vi "rsidr_core_global.vi"() -> ()   [LabVIEW 2020, in "Rohde&Schwarz CMWXP NR FR1 Measurement.lvlib"] (continued)
"Descriptive Name"="Query Multi Eval Meas List EVM DMRS Low Current Limit Check Results", "Data Type"=enum."RawString", "Command"="CALC:NRS:MEAS{instance}:MEV:LIST:MOD:EVM:DMRS:LOW:CURR?", "Access"=enum."Read Only", "Range Table"="", "Read Callback"="", "Write Callback"="", "Range Callback"="", "Check Callback"="", "Rngtable Callback"="", "Coerce Callback"="", "Supported Models"="", "Instrument Options"="", "Check Status Callback"="", "Flags"=0, "Help"="Return error vector magnitude DMRS limit check results for low EVM window position, for all measured list mode segments.\n\nReturn values:  \n<Reliability>\n decimal\n\n<EVM_DMRSLimCheck>\n limit check result\nComma-separated list of values, one per measured segment\nDefault unit:  %\n\nAvailable Repeated Capabilities:\ninstance: i0, i1, i2, i3, i4, i5, i6, i7, i8, i9, i10, i11, i12, i13, i14, i15, i16, i17, i18, i19, i20, i21, i22, i23, i24, i25, i26, i27, i28, i29, i30, i31, i32\r\n\nRemote-control command(s):\nCALCulate:NRSub:MEAS<i>:MEValuation:LIST:MODulation:EVM:DMRS:LOW:CURRent?"}, {"Level"=5, "Class Only"=FALSE, "Identifier"="RSCMWXPNRFR1M_ATTR_QUERY_MULTI_EVAL_MEAS_LIST_EVM_DMRS_LOW_AVERAGE_LIMIT_CHECK_RESULTS", "Descriptive Name"="Query Multi Eval Meas List EVM DMRS Low Average Limit Check Results", "Data Type"=enum."RawString", "Command"="CALC:NRS:MEAS{instance}:MEV:LIST:MOD:EVM:DMRS:LOW:AVER?", "Access"=enum."Read Only", "Range Table"="", "Read Callback"="", "Write Callback"="", "Range Callback"="", "Check Callback"="", "Rngtable Callback"="", "Coerce Callback"="", "Supported Models"="", "Instrument Options"="", "Check Status Callback"="", "Flags"=0, "Help"="Return average error vector magnitude DMRS limit check results for low EVM window position, for all measured list mode segments.\n\nReturn values:  \n<Reliability>\n decimal\n\n<EVM_DMRSLimCheck>\n limit check result\nComma-separated list of values, one per measured segment\nDefault unit:  %\n\nAvailable Repeated Capabilities:\ninstance: i0, i1, i2, i3, i4, i5, i6, i7, i8, i9, i10, i11, i12, i13, i14, i15, i16, i17, i18, i19, i20, i21, i22, i23, i24, i25, i26, i27, i28, i29, i30, i31, i32\r\n\nRemote-control command(s):\nCALCulate:NRSub:MEAS<i>:MEValuation:LIST:MODulation:EVM:DMRS:LOW:AVERage?"}, {"Level"=5, "Class Only"=FALSE, "Identifier"="RSCMWXPNRFR1M_ATTR_QUERY_MULTI_EVAL_MEAS_LIST_EVM_DMRS_LOW_EXTREME_LIMIT_CHECK_RESULTS", "Descriptive Name"="Query Multi Eval Meas List EVM DMRS Low Extreme Limit Check Results", "Data Type"=enum."RawString", "Command"="CALC:NRS:MEAS{instance}:MEV:LIST:MOD:EVM:DMRS:LOW:EXTR?", "Access"=enum."Read Only", "Range Table"="", "Read Callback"="", "Write Callback"="", "Range Callback"="", "Check Callback"="", "Rngtable Callback"="", "Coerce Callback"="", "Supported Models"="", "Instrument Options"="", "Check Status Callback"="", "Flags"=0, "Help"="Return extreme error vector magnitude DMRS limit check results for low EVM window position, for all measured list mode segments.\n\nReturn values:  \n<Reliability>\n decimal\n\n<EVM_DMRSLimCheck>\n limit check result\nComma-separated list of values, one per measured segment\nDefault unit:  %\n\nAvailable Repeated Capabilities:\ninstance: i0, i1, i2, i3, i4, i5, i6, i7, i8, i9, i10, i11, i12, i13, i14, i15, i16, i17, i18, i19, i20, i21, i22, i23, i24, i25, i26, i27, i28, i29, i30, i31, i32\r\n\nRemote-control command(s):\nCALCulate:NRSub:MEAS<i>:MEValuation:LIST:MODulation:EVM:DMRS:LOW:EXTReme?"}, {"Level"=5, "Class Only"=FALSE, "Identifier"="RSCMWXPNRFR1M_ATTR_QUERY_MULTI_EVAL_MEAS_LIST_EVM_DMRS_HIGH_CURRENT_LIMIT_CHECK_RESULTS", "Descriptive Name"="Query Multi Eval Meas List EVM DMRS High Current Limit Check Results", "Data Type"=enum."RawString", "Command"="CALC:NRS:MEAS{instance}:MEV:LIST:MOD:EVM:DMRS:HIGH:CURR?", "Access"=enum."Read Only", "Range Table"="", "Read Callback"="", "Write Callback"="", "Range Callback"="", "Check Callback"="", "Rngtable Callback"="", "Coerce Callback"="", "Supported Models"="", "Instrument Options"="", "Check Status Callback"="", "Flags"=0, "Help"="Return error vector magnitude DMRS limit check results for high EVM window position, for all measured list mode segments.\n\nReturn values:  \n<Reliability>\n decimal\n\n<EVM_DMRSLimCheck>\n limit check result\nComma-separated list of values, one per measured segment\nDefault unit:  %\n\nAvailable Repeated Capabilities:\ninstance: i0, i1, i2, i3, i4, i5, i6, i7, i8, i9, i10, i11, i12, i13, i14, i15, i16, i17, i18, i19, i20, i21, i22, i23, i24, i25, i26, i27, i28, i29, i30, i31, i32\r\n\nRemote-control command(s):\nCALCulate:NRSub:MEAS<i>:MEValuation:LIST:MODulation:EVM:DMRS:HIGH:CURRent?"}, {"Level"=5, "Class Only"=FALSE, "Identifier"="RSCMWXPNRFR1M_ATTR_QUERY_MULTI_EVAL_MEAS_LIST_EVM_DMRS_HIGH_AVERAGE_LIMIT_CHECK_RESULTS", "Descriptive Name"="Query Multi Eval Meas List EVM DMRS High Average Limit Check Results", "Data Type"=enum."RawString", "Command"="CALC:NRS:MEAS{instance}:MEV:LIST:MOD:EVM:DMRS:HIGH:AVER?", "Access"=enum."Read Only", "Range Table"="", "Read Callback"="", "Write Callback"="", "Range Callback"="", "Check Callback"="", "Rngtable Callback"="", "Coerce Callback"="", "Supported Models"="", "Instrument Options"="", "Check Status Callback"="", "Flags"=0, "Help"="Return average error vector magnitude DMRS limit check results for high EVM window position, for all measured list mode segments.\n\nReturn values:  \n<Reliability>\n decimal\n\n<EVM_DMRSLimCheck>\n limit check result\nComma-separated list of values, one per measured segment\nDefault unit:  %\n\nAvailable Repeated Capabilities:\ninstance: i0, i1, i2, i3, i4, i5, i6, i7, i8, i9, i10, i11, i12, i13, i14, i15, i16, i17, i18, i19, i20, i21, i22, i23, i24, i25, i26, i27, i28, i29, i30, i31, i32\r\n\nRemote-control command(s):\nCALCulate:NRSub:MEAS<i>:MEValuation:LIST:MODulation:EVM:DMRS:HIGH:AVERage?"}, {"Level"=5, "Class Only"=FALSE, "Identifier"="RSCMWXPNRFR1M_ATTR_QUERY_MULTI_EVAL_MEAS_LIST_EVM_DMRS_HIGH_EXTREME_LIMIT_CHECK_RESULTS", "Descriptive Name"="Query Multi Eval Meas List EVM DMRS High Extreme Limit Check Results", "Data Type"=enum."RawString", "Command"="CALC:NRS:MEAS{instance}:MEV:LIST:MOD:EVM:DMRS:HIGH:EXTR?", "Access"=enum."Read Only", "Range Table"="", "Read Callback"="", "Write Callback"="", "Range Callback"="", "Check Callback"="", "Rngtable Callback"="", "Coerce Callback"="", "Supported Models"="", "Instrument Options"="", "Check Status Callback"="", "Flags"=0, "Help"="Return extreme error vector magnitude DMRS limit check results for high EVM window position, for all measured list mode segments.\n\nReturn values:  \n<Reliability>\n decimal\n\n<EVM_DMRSLimCheck>\n limit check result\nComma-separated list of values, one per measured segment\nDefault unit:  %\n\nAvailable Repeated Capabilities:\ninstance: i0, i1, i2, i3, i4, i5, i6, i7, i8, i9, i10, i11, i12, i13, i14, i15, i16, i17, i18, i19, i20, i21, i22, i23, i24, i25, i26, i27, i28, i29, i30, i31, i32\r\n\nRemote-control command(s):\nCALCulate:NRSub:MEAS<i>:MEValuation:LIST:MODulation:EVM:DMRS:HIGH:EXTReme?"}, {"Level"=4, "Class Only"=TRUE, "Identifier"="", "Descriptive Name"="Inband Emission", "Data Type"=enum."ViInt32", "Command"="", "Access"=enum."Read Only", "Range Table"="", "Read Callback"="", "Write Callback"="", "Range Callback"="", "Check Callback"="", "Rngtable Callback"="", "Coerce Callback"="", "Supported Models"="", "Instrument Options"="", "Check Status Callback"="", "Flags"=0, "Help"="The attributes in this class return inband emission limit line margin results for all measured segments. The number of returned results depends on the number of measured segments."}, {"Level"=5, "Class Only"=FALSE, "Identifier"="RSCMWXPNRFR1M_ATTR_FETCH_MULTI_EVAL_MEAS_LIST_IEM_MARGIN_CURRENT_RESULTS", "Descriptive Name"="Fetch Multi Eval Meas List IEM Margin Current Results", "Data Type"=enum."RawString", "Command"="FETC:NRS:MEAS{instance}:MEV:LIST:IEM:MARG:CURR?", "Access"=enum."Read Only", "Range Table"="", "Read Callback"="", "Write Callback"="", "Range Callback"="", "Check Callback"="", "Rngtable Callback"="", "Coerce Callback"="", "Supported Models"="", "Instrument Options"="", "Check Status Callback"="", "Flags"=0, "Help"="Return the inband emission limit line margin results for all measured list mode segments. The current margins indicate the minimum (vertical) distance between the limit line and the current trace. A negative result indicates that the limit is exceeded. The average, extreme and standard deviation values are calculated from the current margins.\n\nThe results are returned as triplets per segment: <Reliability>, {<Margin>, <IQImage>, <CarrLeakage>}seg 1, {<Margin>, <IQImage>, <CarrLeakage>}seg 2, ...\n\nReturn values:  \n<Reliability>\n decimal\n\n<Margin>\n float\nMargin over all non-allocated RBs (scope of general limit component)\nDefault unit:  dB \n\n<IQImage>\n float\nMargin at image frequencies of allocated RBs (scope of IQ image limit component)\nDefault unit:  dB \n\n<CarrLeakage>\n float\nMargin at the carrier frequency (scope of IQ offset limit component)\nDefault unit:  dB\n\nAvailable Repeated Capabilities:\ninstance: i0, i1, i2, i3, i4, i5, i6, i7, i8, i9, i10, i11, i12, i13, i14, i15, i16, i17, i18, i19, i20, i21, i22, i23, i24, i25, i26, i27, i28, i29, i30, i31, i32\r\n\nRemote-control command(s):\nFETCh:NRSub:MEAS<i>:MEValuation:LIST:IEMission:MARGin:CURRent?"}, {"Level"=5, "Class Only"=FALSE, "Identifier"="RSCMWXPNRFR1M_ATTR_FETCH_MULTI_EVAL_MEAS_LIST_IEM_MARGIN_AVERAGE_RESULTS", "Descriptive Name"="Fetch Multi Eval Meas List IEM Margin Average Results", "Data Type"=enum."RawString", "Command"="FETC:NRS:MEAS{instance}:MEV:LIST:IEM:MARG:AVER?", "Access"=enum."Read Only", "Range Table"="", "Read Callback"="", "Write Callback"="", "Range Callback"="", "Check Callback"="", "Rngtable Callback"="", "Coerce Callback"="", "Supported Models"="", "Instrument Options"="", "Check Status Callback"="", "Flags"=0, "Help"="Return the average inband emission limit line margin results for all measured list mode segments. The current margins indicate the minimum (vertical) distance between the limit line and the current trace. A negative result indicates that the limit is exceeded. The average, extreme and standard deviation values are calculated from the current margins.\n\nThe results are returned as triplets per segment: <Reliability>, {<Margin>, <IQImage>, <CarrLeakage>}seg 1, {<Margin>, <IQImage>, <CarrLeakage>}seg 2, ...\n\nReturn values:  \n<Reliability>\n decimal\n\n<Margin>\n float\nMargin over all non-allocated RBs (scope of general limit component)\nDefault unit:  dB \n\n<IQImage>\n float\nMargin at image frequencies of allocated RBs (scope of IQ image limit component)\nDefault unit:  dB \n\n<CarrLeakage>\n float\nMargin at the carrier frequency (scope of IQ offset limit component)\nDefault unit:  dB\n\nAvailable Repeated Capabilities:\ninstance: i0, i1, i2, i3, i4, i5, i6, i7, i8, i9, i10, i11, i12, i13, i14, i15, i16, i17, i18, i19, i20, i21, i22, i23, i24, i25, i26, i27, i28, i29, i30, i31, i32\r\n\nRemote-control command(s):\nFETCh:NRSub:MEAS<i>:MEValuation:LIST:IEMission:MARGin:AVERage?"}, {"Level"=5, "Class Only"=FALSE, "Identifier"="RSCMWXPNRFR1M_ATTR_FETCH_MULTI_EVAL_MEAS_LIST_IEM_MARGIN_EXTREME_RESULTS", "Descriptive Name"="Fetch Multi Eval Meas List IEM Margin Extreme Results", "Data Type"=enum."RawString", "Command"="FETC:NRS:MEAS{instance}:MEV:LIST:IEM:MARG:EXTR?", "Access"=enum."Read Only", "Range Table"="", "Read Callback"="", "Write Callback"="", "Range Callback"="", "Check Callback"="", "Rngtable Callback"="", "Coerce Callback"="", "Supported Models"="", "Instrument Options"="", "Check Status Callback"="", "Flags"=0, "Help"="Return the extreme inband emission limit line margin results for all measured list mode segments. The current margins indicate the minimum (vertical) distance between the limit line and the current trace. A negative result indicates that the limit is exceeded. The average, extreme and standard deviation values are calculated from the current margins.\n\nThe results are returned as triplets per segment: <Reliability>, {<Margin>, <IQImage>, <CarrLeakage>}seg 1, {<Margin>, <IQImage>, <CarrLeakage>}seg 2, ...\n\nReturn values:  \n<Reliability>\n decimal\n\n<Margin>\n float\nMargin over all non-allocated RBs (scope of general limit component)\nDefault unit:  dB \n\n<IQImage>\n float\nMargin at image frequencies of allocated RBs (scope of IQ image limit component)\nDefault unit:  dB \n\n<CarrLeakage>\n float\nMargin at the carrier frequency (scope of IQ offset limit component)\nDefault unit:  dB\n\nAvailable Repeated Capabilities:\ninstance: i0, i1, i2, i3, i4, i5, i6, i7, i8, i9, i10, i11, i12, i13, i14, i15, i16, i17, i18, i19, i20, i21, i22, i23, i24, i25, i26, i27, i28, i29, i30, i31, i32\r\n\nRemote-control command(s):\nFETCh:NRSub:MEAS<i>:MEValuation:LIST:IEMission:MARGin:EXTReme?"}, {"Level"=5, "Class Only"=FALSE, "Identifier"="RSCMWXPNRFR1M_ATTR_FETCH_MULTI_EVAL_MEAS_LIST_IEM_MARGIN_STANDARD_DEVIATION_RESULTS", "Descriptive Name"="Fetch Multi Eval Meas List IEM Margin Standard Deviation Results", "Data Type"=enum."RawString", "Command"="FETC:NRS:MEAS{instance}:MEV:LIST:IEM:MARG:SDEV?", "Access"=enum."Read Only", "Range Table"="", "Read Callback"="", "Write Callback"="", "Range Callback"="", "Check Callback"="", "Rngtable Callback"="", "Coerce Callback"="", "Supported Models"="", "Instrument Options"="", "Check Status Callback"="", "Flags"=0, "Help"="Return the standard deviation inband emission limit line margin results for all measured list mode segments. The current margins indicate the minimum (vertical) distance between the limit line and the current trace. A negative result indicates that the limit is exceeded. The average, extreme and standard deviation values are calculated from the current margins.\n\nThe results are returned as triplets per segment: <Reliability>, {<Margin>, <IQImage>, <CarrLeakage>}seg 1, {<Margin>, <IQImage>, <CarrLeakage>}seg 2, ...\n\nReturn values:  \n<Reliability>\n decimal\n\n<Margin>\n float\nMargin over all non-allocated RBs (scope of general limit component)\nDefault unit:  dB \n\n<IQImage>\n float\nMargin at image frequencies of allocated RBs (scope of IQ image limit component)\nDefault unit:  dB \n\n<CarrLeakage>\n float\nMargin at the carrier frequency (scope of IQ offset limit component)\nDefault unit:  dB\n\nAvailable Repeated Capabilities:\ninstance: i0, i1, i2, i3, i4, i5, i6, i7, i8, i9, i10, i11, i12, i13, i14, i15, i16, i17, i18, i19, i20, i21, i22, i23, i24, i25, i26, i27, i28, i29, i30, i31, i32\r\n\nRemote-control command(s):\nFETCh:NRSub:MEAS<i>:MEValuation:LIST:IEMission:MARGin:SDEViation?"}, {"Level"=5, "Class Only"=FALSE, "Identifier"="RSCMWXPNRFR1M_ATTR_FETCH_MULTI_EVAL_MEAS_LIST_IEM_MARGIN_RB_INDEX_CURRENT_RESULTS", "Descriptive Name"="Fetch Multi Eval Meas List IEM Margin RB Index Current Results", "Data Type"=enum."RawString", "Command"="FETC:NRS:MEAS{instance}:MEV:LIST:IEM:MARG:CURR:RBIN?", "Access"=enum."Read Only", "Range Table"="", "Read Callback"="", "Write Callback"="", "Range Callback"="", "Check Callback"="", "Rngtable Callback"="", "Coerce Callback"="", "Supported Models"="", "Instrument Options"="", "Check Status Callback"="", "Flags"=0, "Help"="Return resource block indices of the inband emission measurement for all measured list mode segments. At these RB indices, the current margins have been detected.\n\nThe results are returned as triplets per segment: <Reliability>, {<RBindex>, <IQImage>, <CarrLeakage>}seg 1, {<RBindex>, <IQImage>, <CarrLeakage>}seg 2, ...\n\nReturn values:  \n<Reliability>\n decimal\n\n<RBindex>\n decimal\nResource block index for the general margin (at non-allocated RBs)\n\n<IQImage>\n decimal\nResource block index for the IQ image margin (at image frequencies of allocated RBs)\n\n<CarrLeakage>\n decimal\nResource block index for the carrier leakage margin (at carrier frequency)\n\nAvailable Repeated Capabilities:\ninstance: i0, i1, i2, i3, i4, i5, i6, i7, i8, i9, i10, i11, i12, i13, i14, i15, i16, i17, i18, i19, i20, i21, i22, i23, i24, i25, i26, i27, i28, i29, i30, i31, i32\r\n\nRemote-control command(s):\nFETCh:NRSub:MEAS<i>:MEValuation:LIST:IEMission:MARGin:CURRent:RBINdex?"}, {"Level"=5, "Class Only"=FALSE, "Identifier"="RSCMWXPNRFR1M_ATTR_FETCH_MULTI_EVAL_MEAS_LIST_IEM_MARGIN_RB_INDEX_AVERAGE_RESULTS", "Descriptive Name"="Fetch Multi Eval Meas List IEM Margin RB Index Average Results", "Data Type"=enum."RawString", "Command"="FETC:NRS:MEAS{instance}:MEV:LIST:IEM:MARG:AVER:RBIN?", "Access"=enum."Read Only", "Range Table"="", "Read Callback"="", "Write Callback"="", "Range Callback"="", "Check Callback"="", "Rngtable Callback"="", "Coerce Callback"="", "Supported Models"="", "Instrument Options"="", "Check Status Callback"="", "Flags"=0, "Help"="Return resource block indices of the inband emission measurement for all measured list mode segments. At these RB indices, the average margins have been detected.\n\nThe results are returned as triplets per segment: <Reliability>, {<RBindex>, <IQImage>, <CarrLeakage>}seg 1, {<RBindex>, <IQImage>, <CarrLeakage>}seg 2, ...\n\nReturn values:  \n<Reliability>\n decimal\n\n<RBindex>\n decimal\nResource block index for the general margin (at non-allocated RBs)\n\n<IQImage>\n decimal\nResource block index for the IQ image margin (at image frequencies of allocated RBs)\n\n<CarrLeakage>\n decimal\nResource block index for the carrier leakage margin (at carrier frequency)\n\nAvailable Repeated Capabilities:\ninstance: i0, i1, i2, i3, i4, i5, i6, i7, i8, i9, i10, i11, i12, i13, i14, i15, i16, i17, i18, i19, i20, i21, i22, i23, i24, i25, i26, i27, i28, i29, i30, i31, i32\r\n\nRemote-control command(s):\nFETCh:NRSub:MEAS<i>:MEValuation:LIST:IEMission:MARGin:AVERage:RBINdex?"}, {"Level"=5, "Class Only"=FALSE, "Identifier"="RSCMWXPNRFR1M_ATTR_FETCH_MULTI_EVAL_MEAS_LIST_IEM_MARGIN_RB_INDEX_EXTREME_RESULTS", "Descriptive Name"="Fetch Multi Eval Meas List IEM Margin RB Index Extreme Results", "Data Type"=enum."RawString", "Command"="FETC:NRS:MEAS{instance}:MEV:LIST:IEM:MARG:EXTR:RBIN?", "Access"=enum."Read Only", "Range Table"="", "Read Callback"="", "Write Callback"="", "Range Callback"="", "Check Callback"="", "Rngtable Callback"="", "Coerce Callback"="", "Supported Models"="", "Instrument Options"="", "Check Status Callback"="", "Flags"=0, "Help"="Return extreme resource block indices of the inband emission measurement for all measured list mode segments. At these RB indices, the current margins have been detected.\n\nThe results are returned as triplets per segment: <Reliability>, {<RBindex>, <IQImage>, <CarrLeakage>}seg 1, {<RBindex>, <IQImage>, <CarrLeakage>}seg 2, ...\n\nReturn values:  \n<Reliability>\n decimal\n\n<RBindex>\n decimal\nResource block index for the general margin (at non-allocated RBs)\n\n<IQImage>\n decimal\nResource block index for the IQ image margin (at image frequencies of allocated RBs)\n\n<CarrLeakage>\n decimal\nResource block index for the carrier leakage margin (at carrier frequency)\n\nAvailable Repeated Capabilities:\ninstance: i0, i1, i2, i3, i4, i5, i6, i7, i8, i9, i10, i11, i12, i13, i14, i15, i16, i17, i18, i19, i20, i21, i22, i23, i24, i25, i26, i27, i28, i29, i30, i31, i32\r\n\nRemote-control command(s):\nFETCh:NRSub:MEAS<i>:MEValuation:LIST:IEMission:MARGin:EXTReme:RBINdex?"}, {"Level"=4, "Class Only"=TRUE, "Identifier"="", "Descriptive Name"="Carrier Frequency Error", "Data Type"=enum."ViInt32", "Command"="", "Access"=enum."Read Only", "Range Table"="", "Read Callback"="", "Write Callback"="", "Range Callback"="", "Check Callback"="", "Rngtable Callback"="", "Coerce Callback"="", "Supported Models"="", "Instrument Options"="", "Check Status Callback"="", "Flags"=0, "Help"="The attributes in this class return carrier frequency error results for all measured segments. The number of returned results depends on the number of measured segments."}, {"Level"=5, "Class Only"=FALSE, "Identifier"="RSCMWXPNRFR1M_ATTR_FETCH_MULTI_EVAL_MEAS_LIST_FERR_CURRENT_RESULTS", "Descriptive Name"="Fetch Multi Eval Meas List FERR Current Results", "Data Type"=enum."RawString", "Command"="FETC:NRS:MEAS{instance}:MEV:LIST:MOD:FERR:CURR?", "Access"=enum."Read Only", "Range Table"="", "Read Callback"="", "Write Callback"="", "Range Callback"="", "Check Callback"="", "Rngtable Callback"="", "Coerce Callback"="", "Supported Models"="", "Instrument Options"="", "Check Status Callback"="", "Flags"=0, "Help"="Return carrier frequency error values for all measured list mode segments.\n\nReturn values:  \n<Reliability>\n decimal\n\n<FrequencyError>\n float\nComma-separated list of values, one per measured segment\nDefault unit:  Hz\n\nAvailable Repeated Capabilities:\ninstance: i0, i1, i2, i3, i4, i5, i6, i7, i8, i9, i10, i11, i12, i13, i14, i15, i16, i17, i18, i19, i20, i21, i22, i23, i24, i25, i26, i27, i28, i29, i30, i31, i32\r\n\nRemote-control command(s):\nFETCh:NRSub:MEAS<i>:MEValuation:LIST:MODulation:FERRor:CURRent?"}, {"Level"=5, "Class Only"=FALSE, "Identifier"="RSCMWXPNRFR1M_ATTR_FETCH_MULTI_EVAL_MEAS_LIST_FERR_AVERAGE_RESULTS", "Descriptive Name"="Fetch Multi Eval Meas List FERR Average Results", "Data Type"=enum."RawString", "Command"="FETC:NRS:MEAS{instance}:MEV:LIST:MOD:FERR:AVER?", "Access"=enum."Read Only", "Range Table"="", "Read Callback"="", "Write Callback"="", "Range Callback"="", "Check Callback"="", "Rngtable Callback"="", "Coerce Callback"="", "Supported Models"="", "Instrument Options"="", "Check Status Callback"="", "Flags"=0, "Help"="Return average carrier frequency error values for all measured list mode segments.\n\nReturn values:  \n<Reliability>\n decimal\n\n<FrequencyError>\n float\nComma-separated list of values, one per measured segment\nDefault unit:  Hz\n\nAvailable Repeated Capabilities:\ninstance: i0, i1, i2, i3, i4, i5, i6, i7, i8, i9, i10, i11, i12, i13, i14, i15, i16, i17, i18, i19, i20, i21, i22, i23, i24, i25, i26, i27, i28, i29, i30, i31, i32\r\n\nRemote-control command(s):\nFETCh:NRSub:MEAS<i>:MEValuation:LIST:MODulation:FERRor:AVERage?"}, {"Level"=5, "Class Only"=FALSE, "Identifier"="RSCMWXPNRFR1M_ATTR_FETCH_MULTI_EVAL_MEAS_LIST_FERR_EXTREME_RESULTS", "Descriptive Name"="Fetch Multi Eval Meas List FERR Extreme Results", "Data Type"=enum."RawString", "Command"="FETC:NRS:MEAS{instance}:MEV:LIST:MOD:FERR:EXTR?", "Access"=enum."Read Only", "Range Table"="", "Read Callback"="", "Write Callback"="", "Range Callback"="", "Check Callback"="", "Rngtable Callback"="", "Coerce Callback"="", "Supported Models"="", "Instrument Options"="", "Check Status Callback"="", "Flags"=0, "Help"="Return extreme carrier frequency error values for all measured list mode segments.\n\nReturn values:  \n<Reliability>\n decimal\n\n<FrequencyError>\n float\nComma-separated list of values, one per measured segment\nDefault unit:  Hz\n\nAvailable Repeated Capabilities:\ninstance: i0, i1, i2, i3, i4, i5, i6, i7, i8, i9, i10, i11, i12, i13, i14, i15, i16, i17, i18, i19, i20, i21, i22, i23, i24, i25, i26, i27, i28, i29, i30, i31, i32\r\n\nRemote-control command(s):\nFETCh:NRSub:MEAS<i>:MEValuation:LIST:MODulation:FERRor:EXTReme?"}, {"Level"=5, "Class Only"=FALSE, "Identifier"="RSCMWXPNRFR1M_ATTR_FETCH_MULTI_EVAL_MEAS_LIST_FERR_STANDARD_DEVIATION_RESULTS", "Descriptive Name"="Fetch Multi Eval Meas List FERR Standard Deviation Results", "Data Type"=enum."RawString", "Command"="FETC:NRS:MEAS{instance}:MEV:LIST:MOD:FERR:SDEV?", "Access"=enum."Read Only", "Range Table"="", "Read Callback"="", "Write Callback"="", "Range Callback"="", "Check Callback"="", "Rngtable Callback"="", "Coerce Callback"="", "Supported Models"="", "Instrument Options"="", "Check Status Callback"="", "Flags"=0, "Help"="Return standard deviation carrier frequency error values for all measured list mode segments.\n\nReturn values:  \n<Reliability>\n decimal\n\n<FrequencyError>\n float\nComma-separated list of values, one per measured segment\nDefault unit:  Hz\n\nAvailable Repeated Capabilities:\ninstance: i0, i1, i2, i3, i4, i5, i6, i7, i8, i9, i10, i11, i12, i13, i14, i15, i16, i17, i18, i19, i20, i21, i22, i23, i24, i25, i26, i27, i28, i29, i30, i31, i32\r\n\nRemote-control command(s):\nFETCh:NRSub:MEAS<i>:MEValuation:LIST:MODulation:FERRor:SDEViation?"}, {"Level"=5, "Class Only"=FALSE, "Identifier"="RSCMWXPNRFR1M_ATTR_QUERY_MULTI_EVAL_MEAS_LIST_FERR_CURRENT_LIMIT_CHECK_RESULTS", "Descriptive Name"="Query Multi Eval Meas List FERR Current Limit Check Results", "Data Type"=enum."RawString", "Command"="CALC:NRS:MEAS{instance}:MEV:LIST:MOD:FERR:CURR?", "Access"=enum."Read Only", "Range Table"="", "Read Callback"="", "Write Callback"="", "Range Callback"="", "Check Callback"="", "Rngtable Callback"="", "Coerce Callback"="", "Supported Models"="", "Instrument Options"="", "Check Status Callback"="", "Flags"=0, "Help"="Return carrier frequency error values for all measured list mode segments.\n\nReturn values:  \n<Reliability>\n decimal\n\n<FrequencyErrorLimCheck>\n limit check result\nComma-separated list of values, one per measured segment\n\nAvailable Repeated Capabilities:\ninstance: i0, i1, i2, i3, i4, i5, i6, i7, i8, i9, i10, i11, i12, i13, i14, i15, i16, i17, i18, i19, i20, i21, i22, i23, i24, i25, i26, i27, i28, i29, i30, i31, i32\r\n\nRemote-control command(s):\nCALCulate:NRSub:MEAS<i>:MEValuation:LIST:MODulation:FERRor:CURRent?"}, {"Level"=5, "Class Only"=FALSE, "Identifier"="RSCMWXPNRFR1M_ATTR_QUERY_MULTI_EVAL_MEAS_LIST_FERR_AVERAGE_LIMIT_CHECK_RESULTS", "Descriptive Name"="Query Multi Eval Meas List FERR Average Limit Check Results", "Data Type"=enum."RawString", "Command"="CALC:NRS:MEAS{instance}:MEV:LIST:MOD:FERR:AVER?", "Access"=enum."Read Only", "Range Table"="", "Read Callback"="", "Write Callback"="", "Range Callback"="", "Check Callback"="", "Rngtable Callback"="", "Coerce Callback"="", "Supported Models"="", "Instrument Options"="", "Check Status Callback"="", "Flags"=0, "Help"="Return average carrier frequency error values for all measured list mode segments.\n\nReturn values:  \n<Reliability>\n decimal\n\n<FrequencyErrorLimCheck>\n limit check result\nComma-separated list of values, one per measured segment\n\nAvailable Repeated Capabilities:\ninstance: i0, i1, i2, i3, i4, i5, i6, i7, i8, i9, i10, i11, i12, i13, i14, i15, i16, i17, i18, i19, i20, i21, i22, i23, i24, i25, i26, i27, i28, i29, i30, i31, i32\r\n\nRemote-control command(s):\nCALCulate:NRSub:MEAS<i>:MEValuation:LIST:MODulation:FERRor:AVERage?"}, {"Level"=5, "Class Only"=FALSE, "Identifier"="RSCMWXPNRFR1M_ATTR_QUERY_MULTI_EVAL_MEAS_LIST_FERR_EXTREME_LIMIT_CHECK_RESULTS", "Descriptive Name"="Query Multi Eval Meas List FERR Extreme Limit Check Results", "Data Type"=enum."RawString", "Command"="CALC:NRS:MEAS{instance}:MEV:LIST:MOD:FERR:EXTR?", "Access"=enum."Read Only", "Range Table"="", "Read Callback"="", "Write Callback"="", "Range Callback"="", "Check Callback"="", "Rngtable Callback"="", "Coerce Callback"="", "Supported Models"="", "Instrument Options"="", "Check Status Callback"="", "Flags"=0, "Help"="Return extreme carrier frequency error values for all measured list mode segments.\n\nReturn values:  \n<Reliability>\n decimal\n\n<FrequencyErrorLimCheck>\n limit check result\nComma-separated list of values, one per measured segment\n\nAvailable Repeated Capabilities:\ninstance: i0, i1, i2, i3, i4, i5, i6, i7, i8, i9, i10, i11, i12, i13, i14, i15, i16, i17, i18, i19, i20, i21, i22, i23, i24, i25, i26, i27, i28, i29, i30, i31, i32\r\n\nRemote-control command(s):\nCALCulate:NRSub:MEAS<i>:MEValuation:LIST:MODulation:FERRor:EXTReme?"}, {"Level"=4, "Class Only"=TRUE, "Identifier"="", "Descriptive Name"="IQ Offset", "Data Type"=enum."ViInt32", "Command"="", "Access"=enum."Read Only", "Range Table"="", "Read Callback"="", "Write Callback"="", "Range Callback"="", "Check Callback"="", "Rngtable Callback"="", "Coerce Callback"="", "Supported Models"="", "Instrument Options"="", "Check Status Callback"="", "Flags"=0, "Help"="The attributes in this class return I/Q offset results for all measured segments. The number of returned results depends on the number of measured segments."}, {"Level"=5, "Class Only"=FALSE, "Identifier"="RSCMWXPNRFR1M_ATTR_FETCH_MULTI_EVAL_MEAS_LIST_IQ_OFFSET_CURRENT_RESULTS", "Descriptive Name"="Fetch Multi Eval Meas List IQ Offset Current Results", "Data Type"=enum."RawString", "Command"="FETC:NRS:MEAS{instance}:MEV:LIST:MOD:IQOF:CURR?", "Access"=enum."Read Only", "Range Table"="", "Read Callback"="", "Write Callback"="", "Range Callback"="", "Check Callback"="", "Rngtable Callback"="", "Coerce Callback"="", "Supported Models"="", "Instrument Options"="", "Check Status Callback"="", "Flags"=0, "Help"="Return I/Q origin offset values for all measured list mode segments.\n\nReturn values:  \n<Reliability>\n decimal\n\n<IQOffset>\n float\nComma-separated list of values, one per measured segment\nDefault unit:  dBc\n\nAvailable Repeated Capabilities:\ninstance: i0, i1, i2, i3, i4, i5, i6, i7, i8, i9, i10, i11, i12, i13, i14, i15, i16, i17, i18, i19, i20, i21, i22, i23, i24, i25, i26, i27, i28, i29, i30, i31, i32\r\n\nRemote-control command(s):\nFETCh:NRSub:MEAS<i>:MEValuation:LIST:MODulation:IQOFfset:CURRent?"}, {"Level"=5, "Class Only"=FALSE, "Identifier"="RSCMWXPNRFR1M_ATTR_FETCH_MULTI_EVAL_MEAS_LIST_IQ_OFFSET_AVERAGE_RESULTS", "Descriptive Name"="Fetch Multi Eval Meas List IQ Offset Average Results", "Data Type"=enum."RawString", "Command"="FETC:NRS:MEAS{instance}:MEV:LIST:MOD:IQOF:AVER?", "Access"=enum."Read Only", "Range Table"="", "Read Callback"="", "Write Callback"="", "Range Callback"="", "Check Callback"="", "Rngtable Callback"="", "Coerce Callback"="", "Supported Models"="", "Instrument Options"="", "Check Status Callback"="", "Flags"=0, "Help"="Return average I/Q origin offset values for all measured list mode segments.\n\nReturn values:  \n<Reliability>\n decimal\n\n<IQOffset>\n float\nComma-separated list of values, one per measured segment\nDefault unit:  dBc\n\nAvailable Repeated Capabilities:\ninstance: i0, i1, i2, i3, i4, i5, i6, i7, i8, i9, i10, i11, i12, i13, i14, i15, i16, i17, i18, i19, i20, i21, i22, i23, i24, i25, i26, i27, i28, i29, i30, i31, i32\r\n\nRemote-control command(s):\nFETCh:NRSub:MEAS<i>:MEValuation:LIST:MODulation:IQOFfset:AVERage?"}, {"Level"=5, "Class Only"=FALSE, "Identifier"="RSCMWXPNRFR1M_ATTR_FETCH_MULTI_EVAL_MEAS_LIST_IQ_OFFSET_EXTREME_RESULTS", "Descriptive Name"="Fetch Multi Eval Meas List IQ Offset Extreme Results", "Data Type"=enum."RawString", "Command"="FETC:NRS:MEAS{instance}:MEV:LIST:MOD:IQOF:EXTR?", "Access"=enum."Read Only", "Range Table"="", "Read Callback"="", "Write Callback"="", "Range Callback"="", "Check Callback"="", "Rngtable Callback"="", "Coerce Callback"="", "Supported Models"="", "Instrument Options"="", "Check Status Callback"="", "Flags"=0, "Help"="Return extreme I/Q origin offset values for all measured list mode segments.\n\nReturn values:  \n<Reliability>\n decimal\n\n<IQOffset>\n float\nComma-separated list of values, one per measured segment\nDefault unit:  dBc\n\nAvailable Repeated Capabilities:\ninstance: i0, i1, i2, i3, i4, i5, i6, i7, i8, i9, i10, i11, i12, i13, i14, i15, i16, i17, i18, i19, i20, i21, i22, i23, i24, i25, i26, i27, i28, i29, i30, i31, i32\r\n\nRemote-control command(s):\nFETCh:NRSub:MEAS<i>:MEValuation:LIST:MODulation:IQOFfset:EXTReme?"}, {"Level"=5, "Class Only"=FALSE, "Identifier"="RSCMWXPNRFR1M_ATTR_FETCH_MULTI_EVAL_MEAS_LIST_IQ_OFFSET_STANDARD_DEVIATION_RESULTS", "Descriptive Name"="Fetch Multi Eval Meas List IQ Offset Standard Deviation Results", "Data Type"=enum."RawString", "Command"="FETC:NRS:MEAS{instance}:MEV:LIST:MOD:IQOF:SDEV?", "Access"=enum."Read Only", "Range Table"="", "Read Callback"="", "Write Callback"="", "Range Callback"="", "Check Callback"="", "Rngtable Callback"="", "Coerce Callback"="", "Supported Models"="", "Instrument Options"="", "Check Status Callback"="", "Flags"=0, "Help"="Return standard deviation I/Q origin offset values for all measured list mode segments.\n\nReturn values:  \n<Reliability>\n decimal\n\n<IQOffset>\n float\nComma-separated list of values, one per measured segment\nDefault unit:  dBc\n\nAvailable Repeated Capabilities:\ninstance: i0, i1, i2, i3, i4, i5, i6, i7, i8, i9, i10, i11, i12, i13, i14, i15, i16, i17, i18, i19, i20, i21, i22, i23, i24, i25, i26, i27, i28, i29, i30, i31, i32\r\n\nRemote-control command(s):\nFETCh:NRSub:MEAS<i>:MEValuation:LIST:MODulation:IQOFfset:SDEViation?"}, {"Level"=5, "Class Only"=FALSE, "Identifier"="RSCMWXPNRFR1M_ATTR_QUERY_MULTI_EVAL_MEAS_LIST_IQ_OFFSET_CURRENT_LIMIT_CHECK_RESULTS", "Descriptive Name"="Query Multi Eval Meas List IQ Offset Current Limit Check Results", "Data Type"=enum."RawString", "Command"="CALC:NRS:MEAS{instance}:MEV:LIST:MOD:IQOF:CURR?", "Access"=enum."Read Only", "Range Table"="", "Read Callback"="", "Write Callback"="", "Range Callback"="", "Check Callback"="", "Rngtable Callback"="", "Coerce Callback"="", "Supported Models"="", "Instrument Options"="", "Check Status Callback"="", "Flags"=0, "Help"="Return I/Q origin offset values for all measured list mode segments.\n\nReturn values:  \n<Reliability>\n decimal\n\n<IQOffsetLimCheck>\n limit check result\nComma-separated list of values, one per measured segment\n\nAvailable Repeated Capabilities:\ninstance: i0, i1, i2, i3, i4, i5, i6, i7, i8, i9, i10, i11, i12, i13, i14, i15, i16, i17, i18, i19, i20, i21, i22, i23, i24, i25, i26, i27, i28, i29, i30, i31, i32\r\n\nRemote-control command(s):\nCALCulate:NRSub:MEAS<i>:MEValuation:LIST:MODulation:IQOFfset:CURRent?"}, {"Level"=5, "Class Only"=FALSE, "Identifier"="RSCMWXPNRFR1M_ATTR_QUERY_MULTI_EVAL_MEAS_LIST_IQ_OFFSET_AVERAGE_LIMIT_CHECK_RESULTS", "Descriptive Name"="Query Multi Eval Meas List IQ Offset Average Limit Check Results", "Data Type"=enum."RawString", "Command"="CALC:NRS:MEAS{instance}:MEV:LIST:MOD:IQOF:AVER?", "Access"=enum."Read Only", "Range Table"="", "Read Callback"="", "Write Callback"="", "Range Callback"="", "Check Callback"="", "Rngtable Callback"="", "Coerce Callback"="", "Supported Models"="", "Instrument Options"="", "Check Status Callback"="", "Flags"=0, "Help"="Return average I/Q origin offset values for all measured list mode segments.\n\nReturn values:  \n<Reliability>\n decimal\n\n<IQOffsetLimCheck>\n limit check result\nComma-separated list of values, one per measured segment\n\nAvailable Repeated Capabilities:\ninstance: i0, i1, i2, i3, i4, i5, i6, i7, i8, i9, i10, i11, i12, i13, i14, i15, i16, i17, i18, i19, i20, i21, i22, i23, i24, i25, i26, i27, i28, i29, i30, i31, i32\r\n\nRemote-control command(s):\nCALCulate:NRSub:MEAS<i>:MEValuation:LIST:MODulation:IQOFfset:AVERage?"}, {"Level"=5, "Class Only"=FALSE, "Identifier"="RSCMWXPNRFR1M_ATTR_QUERY_MULTI_EVAL_MEAS_LIST_IQ_OFFSET_EXTREME_LIMIT_CHECK_RESULTS", "Descriptive Name"="Query Multi Eval Meas List IQ Offset Extreme Limit Check Results", "Data Type"=enum."RawString", "Command"="CALC:NRS:MEAS{instance}:MEV:LIST:MOD:IQOF:EXTR?", "Access"=enum."Read Only", "Range Table"="", "Read Callback"="", "Write Callback"="", "Range Callback"="", "Check Callback"="", "Rngtable Callback"="", "Coerce Callback"="", "Supported Models"="", "Instrument Options"="", "Check Status Callback"="", "Flags"=0, "Help"="Return extreme I/Q origin offset values for all measured list mode segments.\n\nReturn values:  \n<Reliability>\n decimal\n\n<IQOffsetLimCheck>\n limit check result\nComma-separated list of values, one per measured segment\n\nAvailable Repeated Capabilities:\ninstance: i0, i1, i2, i3, i4, i5, i6, i7, i8, i9, i10, i11, i12, i13, i14, i15, i16, i17, i18, i19, i20, i21, i22, i23, i24, i25, i26, i27, i28, i29, i30, i31, i32\r\n\nRemote-control command(s):\nCALCulate:NRSub:MEAS<i>:MEValuation:LIST:MODulation:IQOFfset:EXTReme?"}, {"Level"=4, "Class Only"=TRUE, "Identifier"="", "Descriptive Name"="Magnitude Error", "Data Type"=enum."ViInt32", "Command"="", "Access"=enum."Read Only", "Range Table"="", "Read Callback"="", "Write Callback"="", "Range Callback"="", "Check Callback"="", "Rngtable Callback"="", "Coerce Callback"="", "Supported Models"="", "Instrument Options"="", "Check Status Callback"="", "Flags"=0, "Help"="The attributes in this class return magnitude error results for all measured segments. The number of returned results depends on the number of measured segments."}, {"Level"=5, "Class Only"=FALSE, "Identifier"="RSCMWXPNRFR1M_ATTR_FETCH_MULTI_EVAL_MEAS_LIST_MERR_RMS_LOW_CURRENT_RESULTS", "Descriptive Name"="Fetch Multi Eval Meas List MERR RMS Low Current Results", "Data Type"=enum."RawString", "Command"="FETC:NRS:MEAS{instance}:MEV:LIST:MOD:MERR:RMS:LOW:CURR?", "Access"=enum."Read Only", "Range Table"="", "Read Callback"="", "Write Callback"="", "Range Callback"="", "Check Callback"="", "Rngtable Callback"="", "Coerce Callback"="", "Supported Models"="", "Instrument Options"="", "Check Status Callback"="", "Flags"=0, "Help"="Return magnitude error RMS values for low EVM window position, for all measured list mode segments.\n\nReturn values:  \n<Reliability>\n decimal\n\n<MagErrorRMS>\n float\nComma-separated list of values, one per measured segment\nDefault unit:  %\n\nAvailable Repeated Capabilities:\ninstance: i0, i1, i2, i3, i4, i5, i6, i7, i8, i9, i10, i11, i12, i13, i14, i15, i16, i17, i18, i19, i20, i21, i22, i23, i24, i25, i26, i27, i28, i29, i30, i31, i32\r\n\nRemote-control command(s):\nFETCh:NRSub:MEAS<i>:MEValuation:LIST:MODulation:MERRor:RMS:LOW:CURRent?"}, {"Level"=5, "Class Only"=FALSE, "Identifier"="RSCMWXPNRFR1M_ATTR_FETCH_MULTI_EVAL_MEAS_LIST_MERR_RMS_LOW_AVERAGE_RESULTS", "Descriptive Name"="Fetch Multi Eval Meas List MERR RMS Low Average Results", "Data Type"=enum."RawString", "Command"="FETC:NRS:MEAS{instance}:MEV:LIST:MOD:MERR:RMS:LOW:AVER?", "Access"=enum."Read Only", "Range Table"="", "Read Callback"="", "Write Callback"="", "Range Callback"="", "Check Callback"="", "Rngtable Callback"="", "Coerce Callback"="", "Supported Models"="", "Instrument Options"="", "Check Status Callback"="", "Flags"=0, "Help"="Return average magnitude error RMS values for low EVM window position, for all measured list mode segments.\n\nReturn values:  \n<Reliability>\n decimal\n\n<MagErrorRMS>\n float\nComma-separated list of values, one per measured segment\nDefault unit:  %\n\nAvailable Repeated Capabilities:\ninstance: i0, i1, i2, i3, i4, i5, i6, i7, i8, i9, i10, i11, i12, i13, i14, i15, i16, i17, i18, i19, i20, i21, i22, i23, i24, i25, i26, i27, i28, i29, i30, i31, i32\r\n\nRemote-control command(s):\nFETCh:NRSub:MEAS<i>:MEValuation:LIST:MODulation:MERRor:RMS:LOW:AVERage?"}, {"Level"=5, "Class Only"=FALSE, "Identifier"="RSCMWXPNRFR1M_ATTR_FETCH_MULTI_EVAL_MEAS_LIST_MERR_RMS_LOW_EXTREME_RESULTS", "Descriptive Name"="Fetch Multi Eval Meas List MERR RMS Low Extreme Results", "Data Type"=enum."RawString", "Command"="FETC:NRS:MEAS{instance}:MEV:LIST:MOD:MERR:RMS:LOW:EXTR?", "Access"=enum."Read Only", "Range Table"="", "Read Callback"="", "Write Callback"="", "Range Callback"="", "Check Callback"="", "Rngtable Callback"="", "Coerce Callback"="", "Supported Models"="", "Instrument Options"="", "Check Status Callback"="", "Flags"=0, "Help"="Return extreme magnitude error RMS values for low EVM window position, for all measured list mode segments.\n\nReturn values:  \n<Reliability>\n decimal\n\n<MagErrorRMS>\n float\nComma-separated list of values, one per measured segment\nDefault unit:  %\n\nAvailable Repeated Capabilities:\ninstance: i0, i1, i2, i3, i4, i5, i6, i7, i8, i9, i10, i11, i12, i13, i14, i15, i16, i17, i18, i19, i20, i21, i22, i23, i24, i25, i26, i27, i28, i29, i30, i31, i32\r\n\nRemote-control command(s):\nFETCh:NRSub:MEAS<i>:MEValuation:LIST:MODulation:MERRor:RMS:LOW:EXTReme?"}, {"Level"=5, "Class Only"=FALSE, "Identifier"="RSCMWXPNRFR1M_ATTR_FETCH_MULTI_EVAL_MEAS_LIST_MERR_RMS_LOW_STANDARD_DEVIATION_RESULTS", "Descriptive 
